vi "Embedded DB - SET - Actor_Name.vi"(8 "error in (no error)":errorcluster, 10 "Actor_Name IN":string, 11 "Child_6_Class in":refnum<class "Embedded_DB_Class.lvclass">) -> (0 "error out":errorcluster, 2 "Actor Name Out":string, 3 "Child_6_Class out":refnum<class "Embedded_DB_Class.lvclass">)   [LabVIEW 2023, in "Embedded_DB_Actor.lvlib" / "Embedded_DB_Class.lvclass"]
uses:
  Embedded_DB_Class.lvclass
  Embedded_DB_Class.lvclass/Embedded_DB_Class.ctl
  <vilib>/Utility/error.llb/Trim Whitespace One-Sided.vi
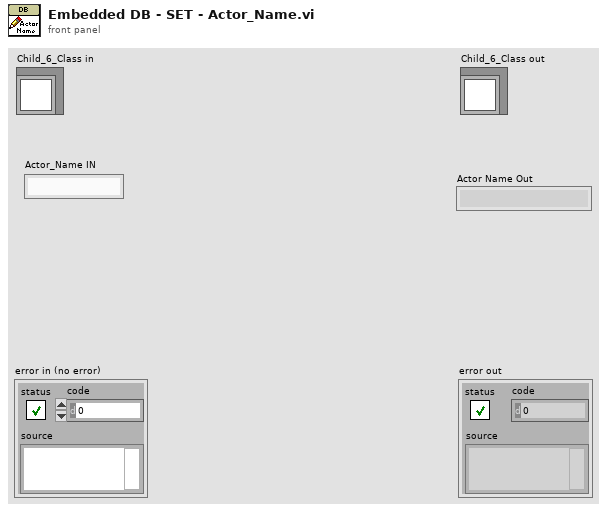
[diagram p1: front panel]
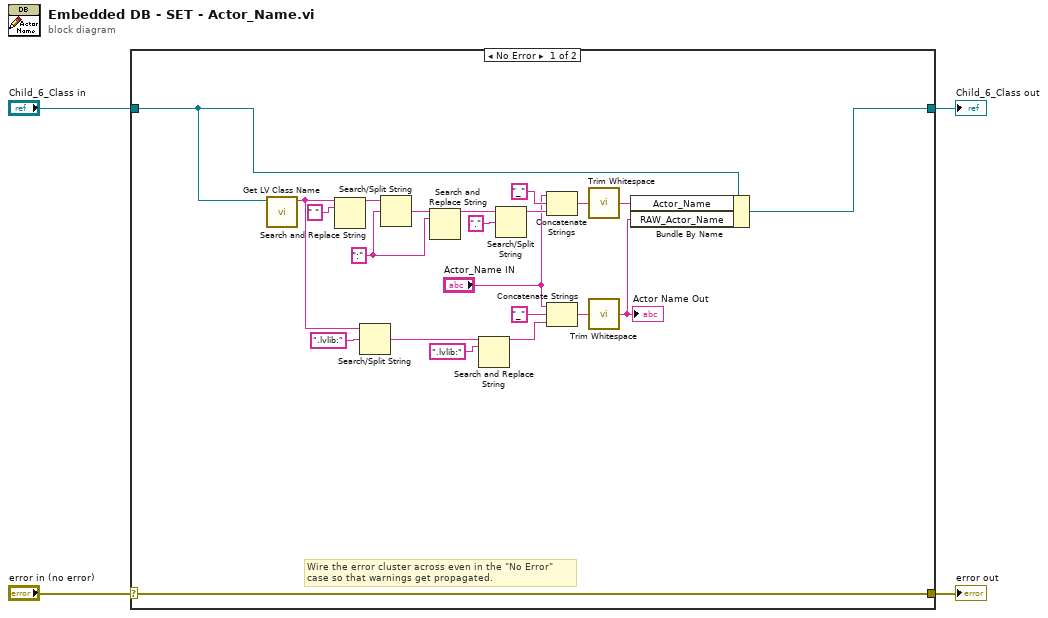
[diagram p0: block diagram]
diagram:
  n1 = case shown="No Error" "error in (no error)" {
    selector: "error in (no error)" -> [w26 w28]
    tunnel: [w26 w28] -> w3
    tunnel: [w5 w27] -> w1
    tunnel: "Child_6_Class in" -> [w6 w27]
    frame No Error {
      w22 = ":" ("search string/char (-)")
      # "Wire the error cluster across even in the \"No Error\"\ncase so that warnings get propagated."
      n2 = call <vilib>:"Get LV Class Name.vi"("object"=w6) -> ("class name"=w12:string)  [unwired: 9 in, 1 out]
      n3 = Search and Replace String(input string=w12, search string=" ") -> (result string=w24:string)  [unwired: 6 in, 3 out]
      n4 = Search/Split String(string=w12, search string/char (-)=".lvlib:") -> (match + rest of string=w15:string)  [unwired: 1 in, 2 out]
      n5 = Search/Split String(string=w24, search string/char (-)=w22) -> (match + rest of string=w23:string)  [unwired: 1 in, 2 out]
      n6 = Search and Replace String(input string=w23, search string=w22) -> (result string=w19:string)  [unwired: 6 in, 3 out]
      n7 = Search and Replace String(input string=w15, search string=".lvlib:" ("search string/char (-)")) -> (result string=w14:string)  [unwired: 6 in, 3 out]
      n8 = Search/Split String(string=w19, search string/char (-)=".") -> (substring before match=w17:string)  [unwired: 1 in, 2 out]
      n9 = Concatenate Strings("Actor_Name IN", "_" ("string"), w17) -> (w20:string)
      n10 = Concatenate Strings("Actor_Name IN", "_" ("string"), w14) -> (w13:string)
      n11 = call <vilib>:"Trim Whitespace.vi"("string"=w20) -> ("trimmed string"=w9:string)  [unwired: 1 in]
      n12 = call <vilib>:"Trim Whitespace.vi"("string"=w13) -> ("trimmed string"=w8:string)  [unwired: 1 in]
      "Actor Name Out" <- w8
      n13 = Bundle By Name(cluster=w6, "Actor_Name"=w9, "RAW_Actor_Name"=w8) -> (w5:refnum<class "Embedded_DB_Class.lvclass">)
    }
    frame Error {
    }
  }
  "error out" <- w3
  "Child_6_Class out" <- w1
